vi "Set Rate for Waveform Stream.vi"   [LabVIEW 2020, in "NI_VS Waveform Streaming Interface.lvlib"]
doc: "Sets whether to stream waveform values at the same rate the device acquires data or at a custom rate you specify. You must manually select the polymorphic instance to use."
uses:
  <vilib>/NI VeriStand/Execution/WaveformStreaming/NI_VS Waveform Streaming Interface.lvlib
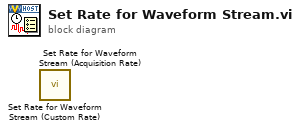
[diagram p0: block diagram]
diagram:
  n1 = call <vilib>:"Set Rate for Waveform Stream (Custom Rate).vi"() -> ()  [unwired: 10 in, 2 out]
  n2 = call <vilib>:"Set Rate for Waveform Stream (Acquisition Rate).vi"() -> ()  [unwired: 10 in, 2 out]
